vi "SeCrTs-Configuration Data.vi"(7 "Enum":enum16{"Read", "Write"}(ring), 8 "error in":errorcluster, 11 "data":T1={"AO config"=[], "AI config"=[], "DI config"=[], "DO config"=[], "TC config"=[], "ACC config"=[], "SG config"=[], "Strain Gauge Settings"={"poisson ratio"=0.0, "nominal gage resistance"=120.0, "gage factor"=2.0}, "Bridge Settings"={"voltage excitation value"=3.0, "voltage excitation source"=10200, "initial bridge voltage"=0.0, "lead wire resistance"=1.7, "strain configuration"=10271}, "Sample Rate"={"AI Sample Rate"=[], "AO Sample Rate"=[], "DI Sample Rate"=[], "TC Sample Rate"=[], "DO Sample Rate"=[], "SG Sample Rate"=[], "ACC Sample Rate"=[]}} {"Bridge Settings"."strain configuration" items=["Full Bridge I"=10183, "Full Bridge II"=10184, "Full Bridge III"=10185, "Half Bridge I"=10188, "Half Bridge II"=10189, "Quarter Bridge I"=10271, "Quarter Bridge II"=10272]; "Bridge Settings"."voltage excitation source" items=["Internal"=10200, "External"=10167, "None"=10230]; "ACC config"."Terminal configuration" items=["default"=-1, "RSE"=10083, "NRSE"=10078, "Differential"=10106, "Pseudodifferential"=12529]; "ACC config"."Sensitivity units" items=["mVolts/g"=12509, "Volts/g"=12510]; "TC config"."type" items=["J"=10072, "K"=10073, "N"=10077, "R"=10082, "S"=10085, "T"=10086, "B"=10047, "E"=10055]; "TC config"."units" items=["Deg C", "Deg F", "Kelvins", "Deg R", "From Custom Scale"]}) -> (0 "error out":errorcluster, 3 "data 2":T1={"AO config"=[], "AI config"=[], "DI config"=[], "DO config"=[], "TC config"=[], "ACC config"=[], "SG config"=[], "Strain Gauge Settings"={"poisson ratio"=0.0, "nominal gage resistance"=120.0, "gage factor"=2.0}, "Bridge Settings"={"voltage excitation value"=3.0, "voltage excitation source"=10200, "initial bridge voltage"=0.0, "lead wire resistance"=1.7, "strain configuration"=10271}, "Sample Rate"={"AI Sample Rate"=[], "AO Sample Rate"=[], "DI Sample Rate"=[], "TC Sample Rate"=[], "DO Sample Rate"=[], "SG Sample Rate"=[], "ACC Sample Rate"=[]}} {"Bridge Settings"."strain configuration" items=["Full Bridge I"=10183, "Full Bridge II"=10184, "Full Bridge III"=10185, "Half Bridge I"=10188, "Half Bridge II"=10189, "Quarter Bridge I"=10271, "Quarter Bridge II"=10272]; "Bridge Settings"."voltage excitation source" items=["Internal"=10200, "External"=10167, "None"=10230]; "ACC config"."Terminal configuration" items=["default"=-1, "RSE"=10083, "NRSE"=10078, "Differential"=10106, "Pseudodifferential"=12529]; "ACC config"."Sensitivity units" items=["mVolts/g"=12509, "Volts/g"=12510]; "TC config"."type" items=["J"=10072, "K"=10073, "N"=10077, "R"=10082, "S"=10085, "T"=10086, "B"=10047, "E"=10055]; "TC config"."units" items=["Deg C", "Deg F", "Kelvins", "Deg R", "From Custom Scale"]})   [LabVIEW 2022 SP3]
uses:
  Controls/SeCrTs-Config.ctl
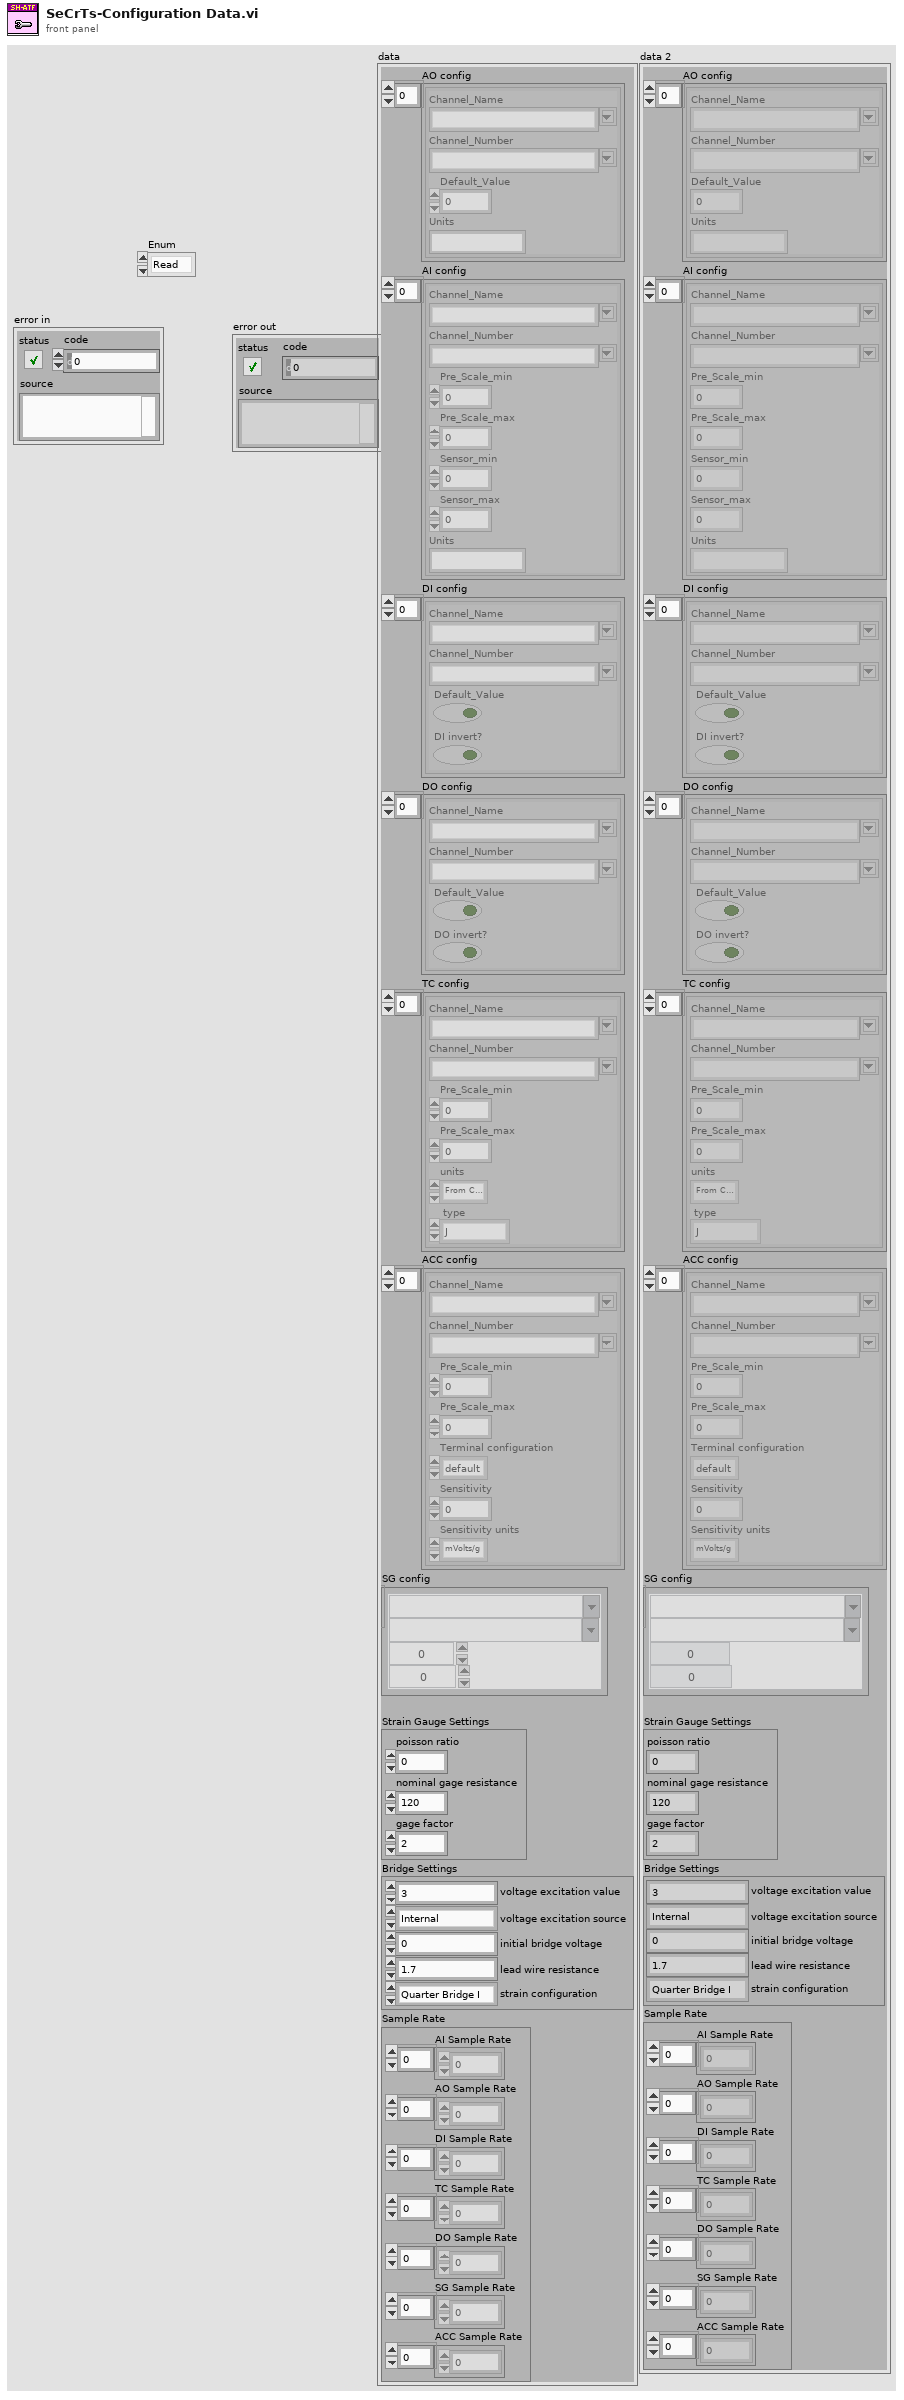
[diagram p1: front panel]
types:
  T1 = typedef "SeCrTs-Config.ctl" = cluster{"AO config":cluster{"Channel_Name":string, "Channel_Number":string, "Default_Value":dbl, "Units":string}[], "AI config":cluster{"Channel_Name":string, "Channel_Number":string, "Pre_Scale_min":dbl, "Pre_Scale_max":dbl, "Sensor_min":dbl, "Sensor_max":dbl, "Units":string}[], "DI config":cluster{"Channel_Name":string, "Channel_Number":string, "Default_Value":bool, "DI invert?":bool}[], "DO config":cluster{"Channel_Name":string, "Channel_Number":string, "Default_Value":bool, "DO invert?":bool}[], "TC config":cluster{"Channel_Name":string, "Channel_Number":string, "Pre_Scale_min":dbl, "Pre_Scale_max":dbl, "units":i32, " type":i32}[], "ACC config":cluster{"Channel_Name":string, "Channel_Number":string, "Pre_Scale_min":dbl, "Pre_Scale_max":dbl, "Terminal configuration":i32, "Sensitivity":dbl, "Sensitivity units":i32}[], "SG config":cluster{"Channel_Name":string, "Channel_Number":string, "Pre_Scale_min":dbl, "Pre_Scale_max":dbl}[], "Strain Gauge Settings":cluster{"poisson ratio":dbl, "nominal gage resistance":dbl, "gage factor":dbl}, "Bridge Settings":cluster{"voltage excitation value":dbl, "voltage excitation source":i32, "initial bridge voltage":dbl, "lead wire resistance":dbl, "strain configuration":i32}, "Sample Rate":cluster{"AI Sample Rate":dbl[], "AO Sample Rate":dbl[], "DI Sample Rate":dbl[], "TC Sample Rate":dbl[], "DO Sample Rate":dbl[], "SG Sample Rate":dbl[], "ACC Sample Rate":dbl[]}}
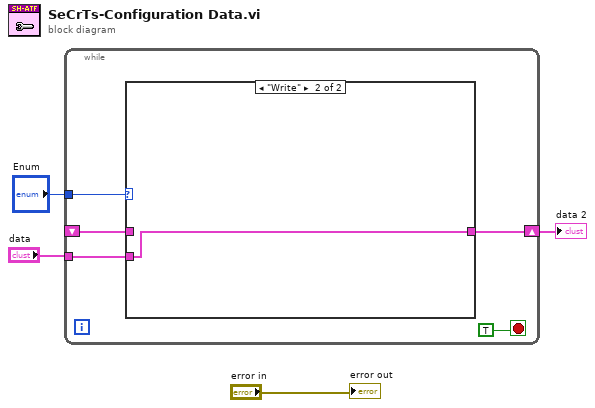
[diagram p0: block diagram]
diagram:
  n1 = while {
    tunnel: "Enum" -> [w9]
    tunnel: "data" -> [w7]
    shift-right: [w6] -> w1
    shift-left: _ -> [w5]
    stop <- TRUE stop-if-true
    n2 = case shown="\"Write\"" w9 {
      tunnel: w7 -> [_ w11]
      tunnel: [w10 w11] -> w6
      tunnel: w5 -> [w10 _]
      frame "Read", Default {
      }
      frame "Write" {
      }
    }
  }
  "data 2" <- w1
  "error out" <- "error in"
